vi "invokenodotnet.vi"   [LabVIEW 2014]
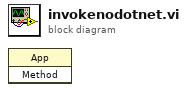
[diagram p0: block diagram]
diagram:
  n1 = invoke class="App" method=#-1() -> ()  [unwired: 3 in, 3 out]
